vi "TestFIFO.vi"() -> ()   [LabVIEW 2013]
panel:
  in  "Fi":dbl
  out "Fo":dbl
  out "Array out":dbl[](array[numeric])
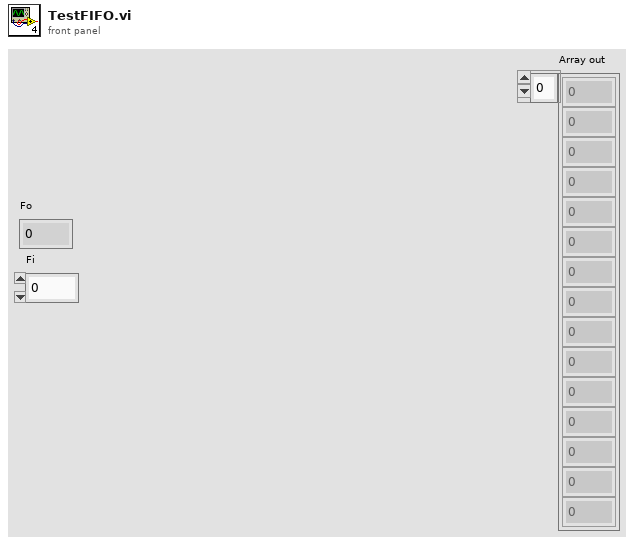
[diagram p1: front panel]
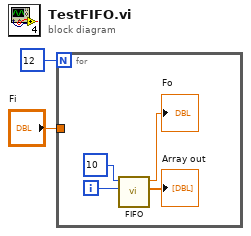
[diagram p0: block diagram]
diagram:
  n1 = for {
    N: 12 -> [_]
    tunnel: "Fi" -> [_]
    i -> [w4]
    n2 = call "FIFO.vi"("Fi"=w4, "FIFO size"=10) -> ("Array out"=→"Array out":dbl[], "Fo"=→"Fo":dbl)  [unwired: 8 in]
  }
